vi "DAQmxChannelsToChannelArray.vi"(11 "DAQmx Physical Channel":tag) -> (3 "Channels Array":string[](array[string]))   [LabVIEW 2016, in "DAQ_Manager.lvclass"]
uses:
  DAQ_Manager.lvclass
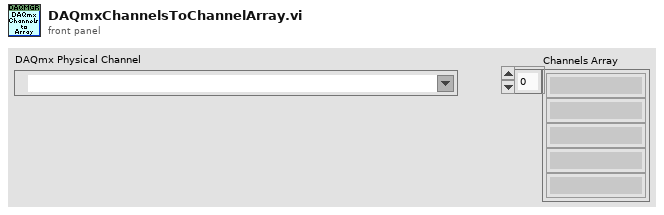
[diagram p1: front panel]
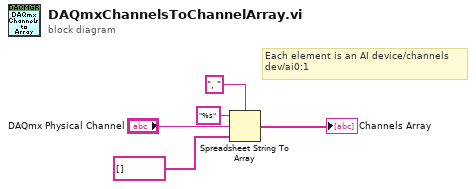
[diagram p0: block diagram]
diagram:
  # "Each element is an AI device/channels\ndev/ai0:1"
  n1 = Spreadsheet String To Array(delimiter (Tab)=", ", format string="%s", spreadsheet string="DAQmx Physical Channel", array type (2D Dbl)=string[] []) -> (array=→"Channels Array":string[])
